vi "GetSetPixelFormat.vi"(7 "Set?":bool, 8 "error in (no error)":errorcluster, 10 "Pixel Format In":string, 11 "Camera in":refnum<class "Camera.lvclass">) -> (0 "error out":errorcluster, 2 "Pixel Format Out":string)   [LabVIEW 2020, in "Camera.lvclass"]
uses:
  Camera.lvclass
  bin/gindustrialcam_32-1.dll
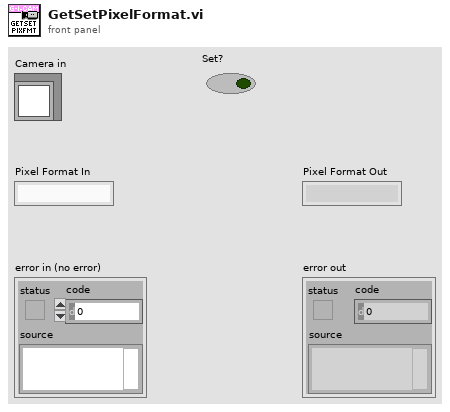
[diagram p1: front panel]
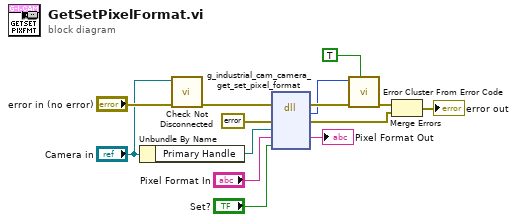
[diagram p0: block diagram]
diagram:
  n1 = Unbundle By Name("Camera in") -> ("Primary Handle"=w3:refnum<data-value>)
  n2 = call "Check Not Disconnected.vi"("error in (no error)"="error in (no error)", "Camera in"="Camera in") -> ("error out"=w2:errorcluster)  [unwired: 9 in]
  n3 = dll-call lib="C:/serenial/lib/g-industrial-camera/LabVIEW/g_industrial_cam/bin/gindustrialcam_*-1.*" fn="g_industrial_cam_camera_get_set_pixel_format"(error in=w2, "err"=errorcluster {"status"=FALSE, "code"=0, "source"=""} ("error constant"), "edvr"=w3, "formats"="Pixel Format In", "set"="Set?") -> (error out=w14:errorcluster, "Mg_Error"=w13:i32, "err"=w11:errorcluster, "formats"=→"Pixel Format Out":string)  [unwired: 4 in, 1 out]
  n4 = call <vilib>:"Error Cluster From Error Code.vi"("show call chain? (False)"=TRUE, "error in (no error)"=w14, "error code (0)"=w13) -> ("error out"=w12:errorcluster)  [unwired: 6 in]
  n5 = Merge Errors(w12, w11) -> (→"error out":errorcluster)
